vi "main.vi"() -> ()   [LabVIEW 2018]
uses:
  cell.ctl
  guess.ctl
panel:
  out "solver array":cluster{"solved":bool, "values":string[]}[][](array[cluster])
  out "puzzle":string[][](array[string])
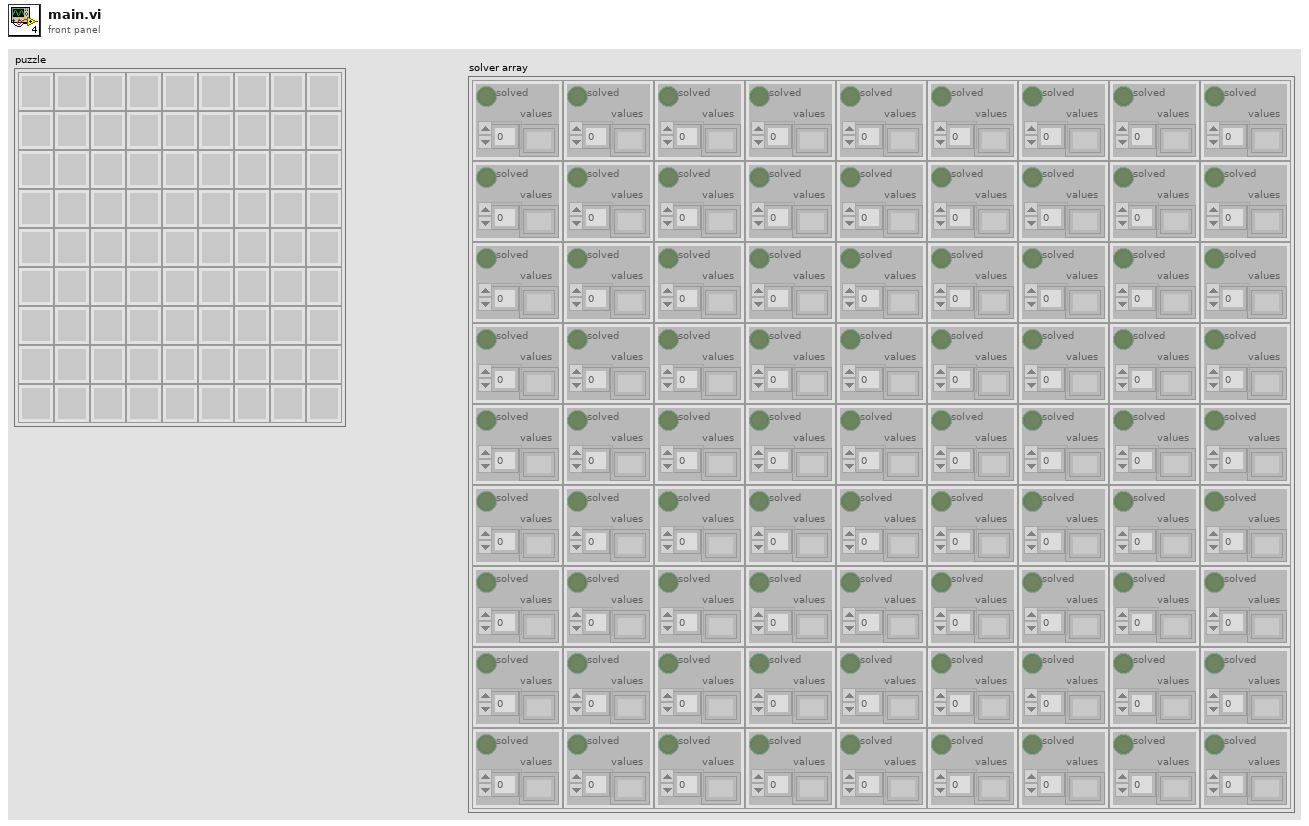
[diagram p1: front panel]
types:
  T1 = typedef "guess.ctl" = cluster{"cell position":cluster{"row":i32, "col":i32}, "guess":string}
  T2 = typedef "cell.ctl" = cluster{"solved":bool, "values":string[]}
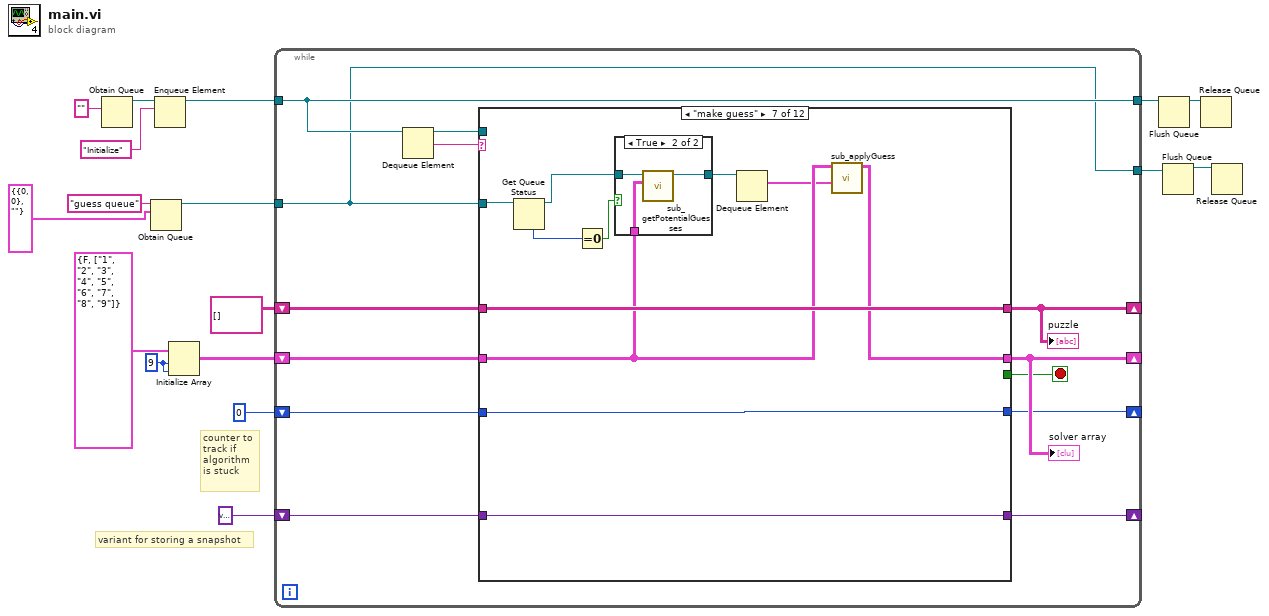
[diagram p0: block diagram]
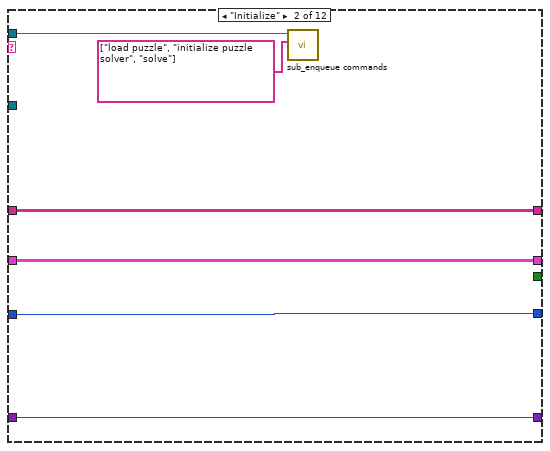
[diagram p3: hidden frame]
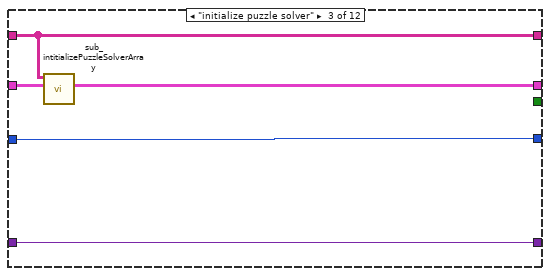
[diagram p4: hidden frame]
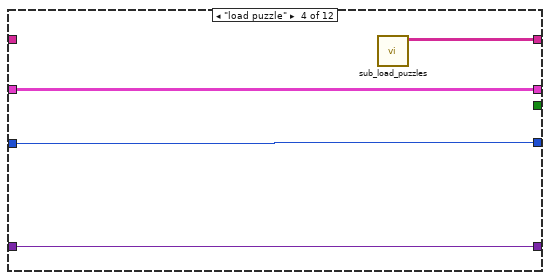
[diagram p5: hidden frame]
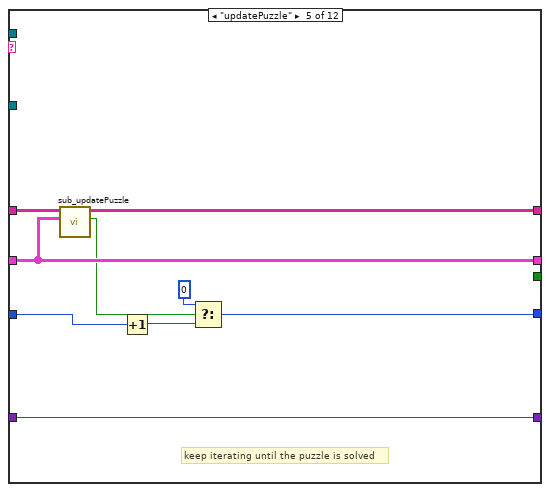
[diagram p6: hidden frame]
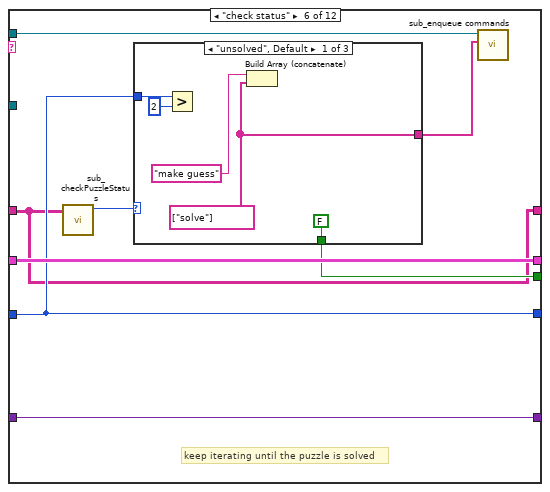
[diagram p7: hidden frame]
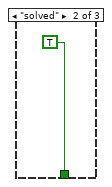
[diagram p8: hidden frame]
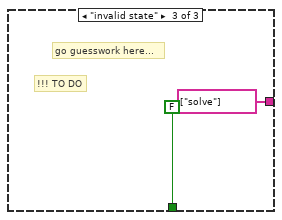
[diagram p9: hidden frame]
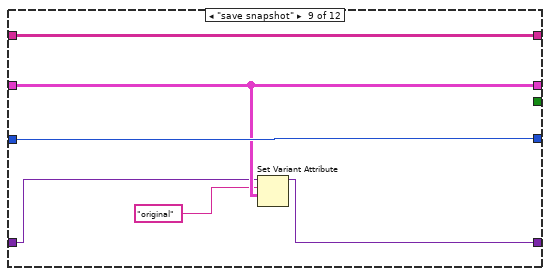
[diagram p12: hidden frame]
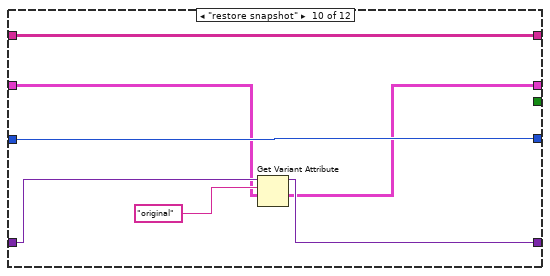
[diagram p13: hidden frame]
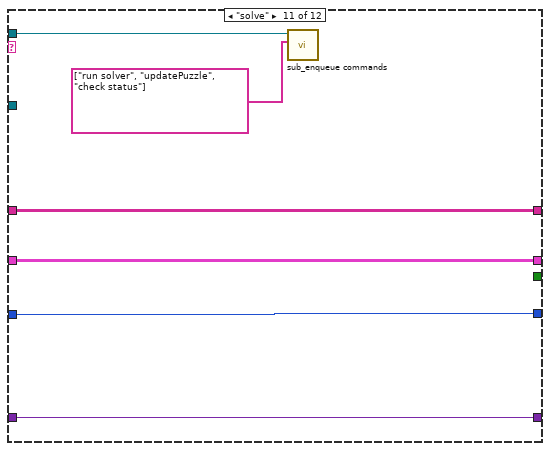
[diagram p14: hidden frame]
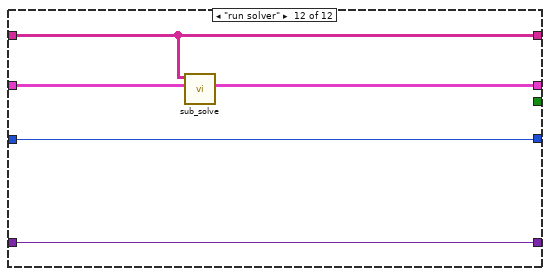
[diagram p15: hidden frame]
diagram:
  w13 = 9 ("dimension size")
  # "variant for storing a snapshot"
  # "counter to\ntrack if \nalgorithm\nis stuck"
  n1 = Obtain Queue(element data type="") -> (queue out=w16:refnum<queue>)  [unwired: 4 in, 2 out]
  n2 = Obtain Queue(name (unnamed)="guess queue", element data type=T1 {"cell position"={"row"=0, "col"=0}, "guess"=""} ("guess")) -> (queue out=w3:refnum<queue>)  [unwired: 3 in, 2 out]
  n3 = Enqueue Element(queue=w16, element="Initialize") -> (queue out=w14:refnum<queue>)  [unwired: 2 in, 2 out]
  n4 = Initialize Array(T2 {"solved"=FALSE, "values"=["1", "2", "3", "4", "5", "6", "7", "8", "9"]} ("cell"), w13, w13) -> (w12:T2[][])
  n5 = while {
    tunnel: w14 -> [w26]
    tunnel: [w26] -> w9
    shift-right: [w25] -> _
    shift-left: w12 -> [w27]
    shift-right: [w24] -> _
    shift-left: string[][] [] ("puzzles (out)") -> [w28]
    shift-right: [w23] -> _
    shift-left: 0 -> [w21]
    shift-right: [w19] -> _
    shift-left: variant -> [w20]
    tunnel: w3 -> [w18]
    tunnel: [w18] -> w2
    stop <- w22 stop-if-true
    n6 = Dequeue Element(queue=w26) -> (queue out=w29:refnum<queue>, element=w30:string)  [unwired: 2 in, 2 out]
    n7 = case shown="\"make guess\"" w30 {
      tunnel: w29 -> [_ w40 _ _ _ w65 _ _ _ _ w110 _]
      tunnel: [w34 w38 w45 w49 w57 w61 w84 w92 w98 w105 w109 w115] -> w24
      tunnel: w28 -> [w34 w38 w45 _ w56 w61 w84 w92 w98 w105 w109 w115]
      tunnel: w27 -> [w33 w37 w44 w48 w58 w66 w77 w91 w97 w101 w112 w116]
      tunnel: [w33 w37 w43 w48 w58 w66 w75 w91 w97 w100 w112 w114] -> w25
      tunnel: w21 -> [w32 w36 w42 w47 w55 w62 w85 w93 w99 w106 w108 w117]
      tunnel: [w32 w36 w42 w47 w51 w62 w85 w93 w99 w106 w108 w117] -> w23
      tunnel: [_ _ _ _ _ w63 _ _ _ _ _ _] -> w22
      tunnel: w20 -> [w31 w35 w41 w46 w50 w59 w83 w90 w96 w104 w107 w113]
      tunnel: [w31 w35 w41 w46 w50 w59 w83 w90 w95 w103 w107 w113] -> w19
      tunnel: w18 -> [_ _ _ _ _ _ w82 _ _ _ _ _]
      frame "False", Default {
      }
      frame "Initialize" {
        n8 = call "sub_enqueue commands.vi"("commands"=string[] ["load puzzle", "initialize puzzle solver", "solve"], "Queue in"=w40) -> ()  [unwired: 10 in]
      }
      frame "initialize puzzle solver" {
        n9 = call "sub_intitializePuzzleSolverArray.vi"("solver array"=w44, "puzzle (in)"=w45) -> ("solver array 2"=w43:cluster{"solved":bool, "values":string[]}[][])  [unwired: 8 in, 1 out]
      }
      frame "load puzzle" {
        n10 = call "sub_load_puzzles.vi"() -> ("puzzles (out)"=w49:string[][])  [unwired: 10 in, 1 out]
      }
      frame "updatePuzzle" {
        # "keep iterating until the puzzle is solved"
        n11 = call "sub_updatePuzzle.vi"("solver array"=w58, "puzzle (in)"=w56) -> ("changes made ?"=w54:bool, "puzzle (out)"=w57:string[][])  [unwired: 7 in, 1 out]
        n12 = Increment(x=w55) -> (x+1=w53:i32)
        n13 = Select(t=0, s=w54, f=w53) -> (s? t:f=w51:i32)
      }
      frame "check status" {
        # "keep iterating until the puzzle is solved"
        n14 = call "sub_checkPuzzleStatus.vi"("puzzle (in)"=w61) -> ("status"=w64:enum16{"unsolved", "solved", "invalid state"})  [unwired: 9 in, 1 out]
        n15 = case shown="\"unsolved\", Default" w64 {
          tunnel: [FALSE TRUE FALSE] -> w63
          tunnel: w62 -> [w70 _ _]
          tunnel: [w67 _ string[] ["solve"] ("commands")] -> w60
          frame "unsolved", Default {
            w67 = string[] ["solve"] ("commands")
            n16 = Greater?(x=w70, y=2) -> ()  [unwired: 1 out]
            n17 = Build Array (concatenate)("make guess", w67) -> ()  [unwired: 1 out]
          }
          frame "solved" {
          }
          frame "invalid state" {
            # "!!! TO DO"
            # "go guesswork here..."
          }
        }
        n18 = call "sub_enqueue commands.vi"("commands"=w60, "Queue in"=w65) -> ()  [unwired: 10 in]
      }
      frame "make guess" {
        n19 = Get Queue Status(queue=w82) -> (queue out=w79:refnum<queue>, # elements in queue=w81:i32)  [unwired: 2 in, 6 out]
        n20 = Equal To 0?(x=w81) -> (x = 0?=w80:bool)
        n21 = case shown="True" w80 {
          tunnel: w77 -> [_ w88]
          tunnel: w79 -> [w86 w89]
          tunnel: [w86 w87] -> w78
          frame False {
          }
          frame True {
            n22 = call "sub_getPotentialGuesses.vi"("solver array"=w88, "guess queue (in)"=w89) -> ("guess queue (out)"=w87:refnum<queue>)  [unwired: 9 in]
          }
        }
        n23 = Dequeue Element(queue=w78) -> (element=w76:T1)  [unwired: 2 in, 3 out]
        n24 = call "sub_applyGuess.vi"("guess"=w76, "solver (in)"=w77) -> ("solver (out)"=w75:T2[][])  [unwired: 9 in]
      }
      frame "undo guess" {
      }
      frame "save snapshot" {
        n25 = Set Variant Attribute(Variant=w96, name="original", value=w97) -> (Variant out=w95:variant)  [unwired: 1 in, 2 out]
      }
      frame "restore snapshot" {
        n26 = Get Variant Attribute(Variant=w104, name="original", default value (empty Variant)=w101) -> (duplicate Variant=w103:variant, value=w100:T2[][])  [unwired: 1 in, 2 out]
      }
      frame "solve" {
        n27 = call "sub_enqueue commands.vi"("commands"=string[] ["run solver", "updatePuzzle", "check status"], "Queue in"=w110) -> ()  [unwired: 10 in]
      }
      frame "run solver" {
        n28 = call "sub_solve.vi"("solver (in)"=w116, "puzzle (in)"=w115) -> ("solver (out)"=w114:cluster{"solved":bool, "values":string[]}[][])  [unwired: 9 in]
      }
    }
    "puzzle" <- w24
    "solver array" <- w25
  }
  n29 = Flush Queue(queue=w9) -> (queue out=w8:refnum<queue>)  [unwired: 1 in, 2 out]
  n30 = Flush Queue(queue=w2) -> (queue out=w1:refnum<queue>)  [unwired: 1 in, 2 out]
  n31 = Release Queue(queue=w8) -> ()  [unwired: 2 in, 3 out]
  n32 = Release Queue(queue=w1) -> ()  [unwired: 2 in, 3 out]
